vi "ThisDate.vi"() -> (0 "this.Date":string)   [LabVIEW 2023]
uses:
  <vilib>/Utility/file.llb/Read Delimited Spreadsheet (string).vi
panel:
  out "String":string
  out "all rows":string[](array[string])
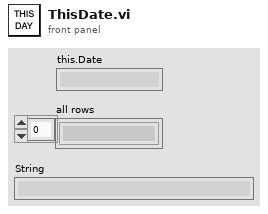
[diagram p1: front panel]
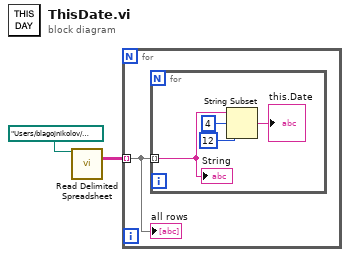
[diagram p0: block diagram]
diagram:
  n1 = call-poly <vilib>:"Read Delimited Spreadsheet.vi"("file path (dialog if empty)"=path "/Users/blagojnikolov/Desktop/@tmp/fromSite.txt" ("file (use dialog)")) -> ("all rows"=w1:string[][])  [unwired: 9 in, 5 out]
  n2 = for {
    tunnel: w1 -> [w3] mode=indexing
    n3 = for {
      tunnel: w3 -> [w7] mode=indexing
      n4 = String Subset(string=w7, offset (0)=4, length (rest)=12 ("length (rest)")) -> (substring=→"this.Date":string)
      "String" <- w7
    }
    "all rows" <- w3
  }
